vi "box.vi"(0 "Box":cluster{"Length":sgl, "Width":sgl, "Height":sgl}={"Length"=1.0, "Width"=1.0, "Height"=1.0}) -> (4 "urdf out":string="<box>\n  <size>1.00 1.00 1.00</size>\n</box>")   [LabVIEW 2012]
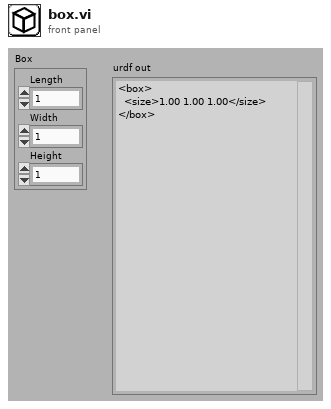
[diagram p1: front panel]
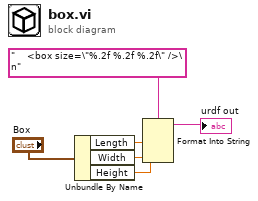
[diagram p0: block diagram]
diagram:
  n1 = Unbundle By Name("Box") -> ("Length"=w4:sgl, "Width"=w3:sgl, "Height"=w1:sgl)
  n2 = Format Into String(format string="    <box size=\"%.2f %.2f %.2f\" />\n", w4, w3, w1) -> (resulting string=→"urdf out":string)  [unwired: 2 in, 1 out]
